vi "myRIO__TCP_constants_byteRange_delim.vi"() -> (2 "output_delim_byte":u8=44, 3 "output_delim_char":string=",")   [LabVIEW 2014]
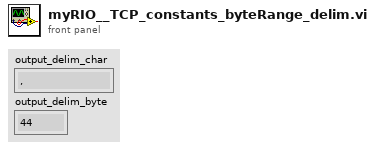
[diagram p1: front panel]
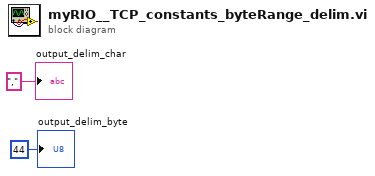
[diagram p0: block diagram]
diagram:
  "output_delim_char" <- ","
  "output_delim_byte" <- u8 44
